vi "runHWLoop.vi"(8 "error in (no error)":errorcluster, 11 "HWController in":refnum<class "HWController.lvclass">) -> (0 "error out":errorcluster, 3 "HWController out":refnum<class "HWController.lvclass">)   [LabVIEW 2009, in "Hardware.lvlib" / "HWControllers.lvlib" / "HWController.lvclass"]
uses:
  HWController.lvclass
  HWController.lvclass/HWController.ctl
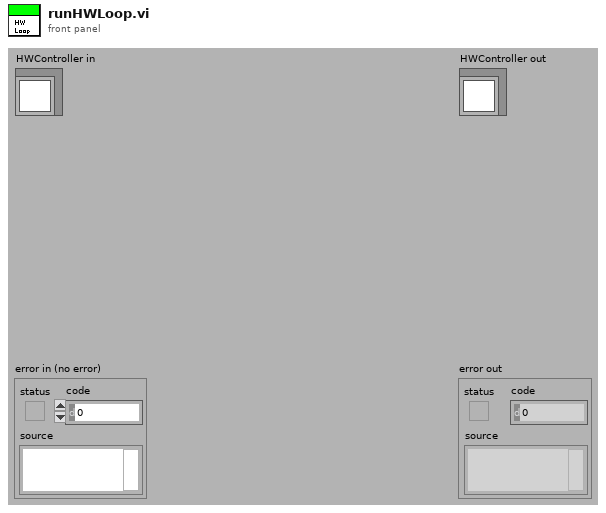
[diagram p1: front panel]
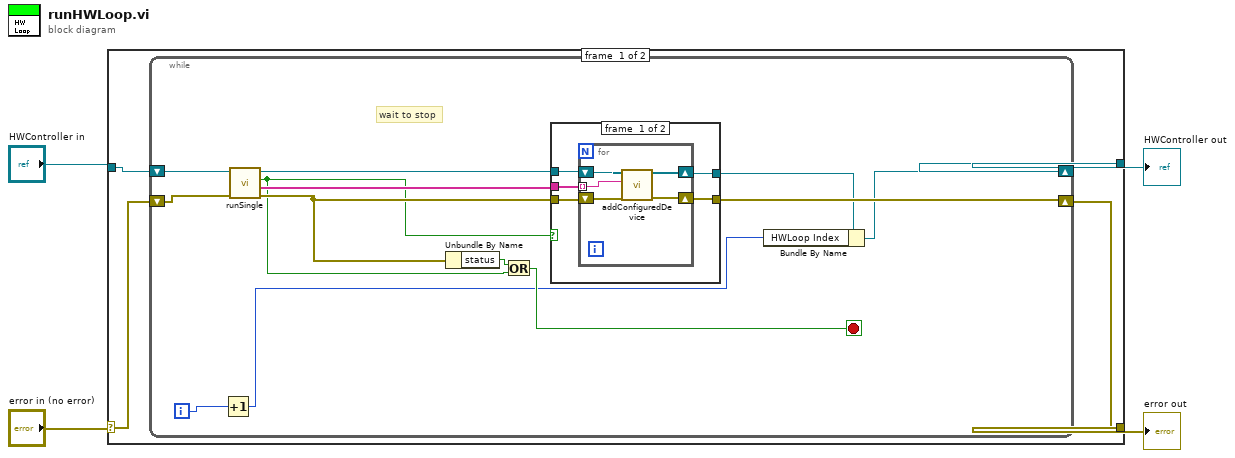
[diagram p0: block diagram]
diagram:
  n1 = case shown="No Error" "error in (no error)" {
    selector: "error in (no error)" -> [w7 w35]
    tunnel: [w5 w35] -> w3
    tunnel: [w6 w34] -> w1
    tunnel: "HWController in" -> [w8 w34]
    frame #0 {
      n2 = while {
        shift-right: [w15] -> w6
        shift-left: w8 -> [w14]
        shift-right: [w19] -> w5
        shift-left: w7 -> [w13]
        i -> [w17]
        stop <- w20 stop-if-true
        # "wait to stop"
        n3 = Increment(x=w17) -> (x+1=w16:i32)
        n4 = call "runSingle.vi"("error in (no error)"=w13, "HWController in"=w14) -> ("error out"=w11:errorcluster, "devicesConfigured"=w10:string[], "Stopped"=w9:bool, "HWController out"=w12:refnum<class "HWController.lvclass">)  [unwired: 6 in]
        n5 = Unbundle By Name(w11) -> ("status"=w21:bool)
        n6 = Or(x=w21, y=w9) -> (x .or. y?=w20:bool)
        n7 = case shown="False" w9 {
          tunnel: w12 -> [w23 w33]
          tunnel: [w24 w33] -> w18
          tunnel: w11 -> [w22 w32]
          tunnel: [w26 w32] -> w19
          tunnel: w10 -> [w25 _]
          frame #0 {
            n8 = for {
              shift-right: [w30] -> w24
              shift-left: w23 -> [w31]
              shift-right: [w29] -> w26
              shift-left: w22 -> [w28]
              tunnel: w25 -> [w27] mode=indexing
              n9 = call "addConfiguredDevice.vi"("error in (no error)"=w28, "deviceName"=w27, "HWController in"=w31) -> ("error out"=w29:errorcluster, "HWController out"=w30:refnum<class "HWController.lvclass">)  [unwired: 7 in]
            }
          }
          frame #1 {
          }
        }
        n10 = Bundle By Name(cluster=w18, "HWLoop Index"=w16) -> (w15:refnum<class "HWController.lvclass">)
      }
    }
    frame #1 {
    }
  }
  "error out" <- w3
  "HWController out" <- w1
